vi "Initialize.vi"(8 "error in (no error)":errorcluster, 11 "MB in":refnum<class "Modbus Master CR.lvclass">) -> (0 "error out":errorcluster, 3 "MB out":refnum<class "Modbus Master CR.lvclass">)   [LabVIEW 2021, in "Modbus Master CR.lvclass"]
uses:
  Modbus Master CR.lvclass
  Modbus Master CR.lvclass/Modbus Master CR.ctl
  Transmission Data Unit/Transmission Data Unit.lvclass
  Data Model/Device Data Model.lvclass
  Network Master/Network Master.lvclass
  C:/my_projects/projects/Algorithms/Labview/21/Modbus_v121c/Network Protocol/Network Master/Network Master.lvclass
  C:/my_projects/projects/Algorithms/Labview/21/Modbus_v121c/Network Protocol/Network Protocol.lvclass
  C:/my_projects/projects/Algorithms/Labview/21/Modbus_v121c/Network Protocol/MB/Modbus Master CR.lvclass
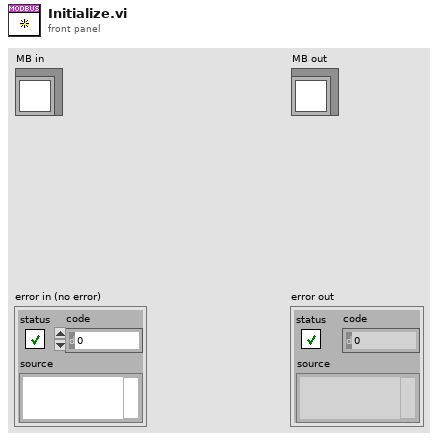
[diagram p1: front panel]
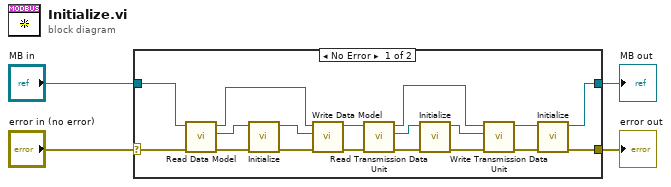
[diagram p0: block diagram]
diagram:
  n1 = case shown="No Error" "error in (no error)" {
    selector: "error in (no error)" -> [w14 w23]
    tunnel: [w17 w23] -> w3
    tunnel: [w16 w24] -> w1
    tunnel: "MB in" -> [w15 w24]
    frame No Error {
      n2 = call "Read Data Model.vi"("error in (no error)"=w14, "MB_TCP in"=w15) -> ("error out"=w21:errorcluster, "Data Model"=w22:refnum<class "Device Data Model.lvclass">, "MB_TCP out"=w18:refnum<class "Modbus Master CR.lvclass">)  [unwired: 7 in]
      n3 = call-dynamic "Initialize.vi"("error in"=w21, "device data model in"=w22) -> ("error out"=w20:errorcluster, "device data model out"=w19:refnum<class "Device Data Model.lvclass">)  [unwired: 8 in]
      n4 = call "Write Data Model.vi"("error in (no error)"=w20, "Data Model"=w19, "MB_TCP in"=w18) -> ("error out"=w12:errorcluster, "MB_TCP out"=w13:refnum<class "Modbus Master CR.lvclass">)  [unwired: 7 in]
      n5 = call "Read Transmission Data Unit.vi"("error in (no error)"=w12, "Network Master in"=w13) -> ("error out"=w10:errorcluster, "Transmission Data Unit"=w11:refnum<class "Transmission Data Unit.lvclass">, "Network Master out"=w7:refnum<class "Modbus Master CR.lvclass">)  [unwired: 7 in]
      n6 = call-dynamic "Initialize.vi"("error in"=w10, "transmission data unit in"=w11) -> ("error out"=w9:errorcluster, "transmission data unit out"=w8:refnum<class "Transmission Data Unit.lvclass">)  [unwired: 8 in]
      n7 = call "Write Transmission Data Unit.vi"("error in (no error)"=w9, "Transmission Data Unit"=w8, "Network Master in"=w7) -> ("error out"=w5:errorcluster, "Network Master out"=w6:refnum<class "Modbus Master CR.lvclass">)  [unwired: 7 in]
      n8 = call-parent "Initialize.vi"("error in"=w5, "Network Master in"=w6) -> ("error out"=w17:errorcluster, "Network Master out"=w16:refnum<class "Modbus Master CR.lvclass">)  [unwired: 8 in]
    }
    frame Error {
    }
  }
  "error out" <- w3
  "MB out" <- w1
